vi "Parse ACL.vi"(11 "String":string) -> (3 "Signed identifiers":T1[](array[typedef]))   [LabVIEW 2015, in "NI_Azure_Blob.lvlib"]
uses:
  NI_Azure_Blob.lvlib
  Signed Identifier.ctl
  Access Policy.ctl
  XML Parsing/NI_Azure_XML Parsing.lvlib
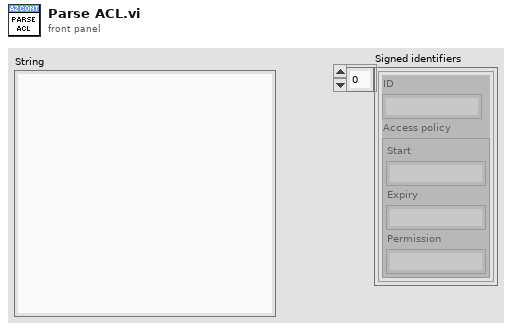
[diagram p1: front panel]
types:
  T1 = typedef "NI_Azure_Blob.lvlib/Signed Identifier.ctl" = cluster{"ID":string, "Access policy":T2}
  T2 = typedef "NI_Azure_Blob.lvlib/Access Policy.ctl" = cluster{"Start":string, "Expiry":string, "Permission":string}
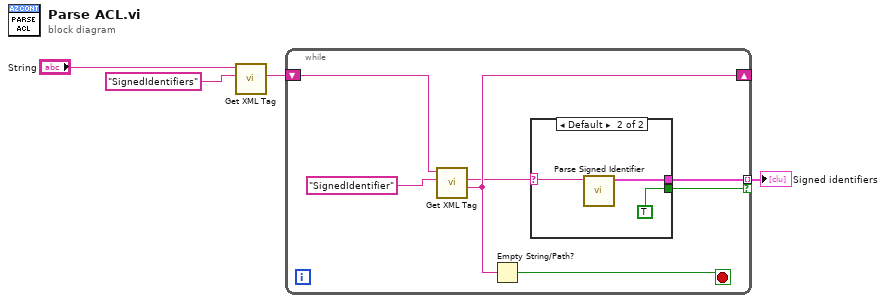
[diagram p0: block diagram]
diagram:
  n1 = call "Get XML Tag.vi"("Tag name"="SignedIdentifiers", "XML String in"="String") -> ("Tag value"=w2:string)  [unwired: 5 in, 4 out]
  n2 = while {
    shift-right: [w8] -> _
    shift-left: w2 -> [w10]
    tunnel: [w6] -> w1 mode=indexing if=w5
    stop <- w9 stop-if-true
    n3 = call "Get XML Tag.vi"("Tag name"="SignedIdentifier", "XML String in"=w10) -> ("Remaining string"=w8:string, "Tag value"=w7:string)  [unwired: 5 in, 3 out]
    n4 = Empty String/Path?(string/path=w8) -> (empty?=w9:bool)
    n5 = case shown="Default" w7 {
      selector: w7 -> [_ w14]
      tunnel: [_ w13] -> w6
      tunnel: [_ TRUE] -> w5
      frame "" {
      }
      frame Default {
        n6 = call "Parse Signed Identifier.vi"("String"=w14) -> ("Signed identifier"=w13:T1)  [unwired: 10 in]
      }
    }
  }
  "Signed identifiers" <- w1
